vi "loginSession.vi"(8 "error in (no error)":errorcluster, 10 "Device index":i32, 11 "SM1000-control in":T1) -> (0 "error out":errorcluster, 3 "SM1000-control out":T1)   [LabVIEW 2013, in "HardwareCharacterization.lvlib" / "HC-SM1000.lvclass"]
doc: "Connect to an EC device by establishing a session.\n\nOnce EC1000 modules have been identified via the use of the Broadcast API, a communications session can be opened between the client an a selected target EC1000. Sessions are established via a call to this method. Multiple sessions to different target EC1000 controllers are made by instantiating separate Session objects. A target EC1000 controller may only serve one client session at a time."
uses:
  HC-SM1000.lvclass
  Object-reference.ctl
  HC-SM1000.lvclass/HC-SM1000.ctl
  Custom-errors.ctl
  C:/Users/vangeste/Desktop/2015-05-29 - SLM - MAIF/HC-HardwareCharacterization/Sources/SM1000/LECSession.dll
  LECSession.dll
  DOTNET-error-int.vi
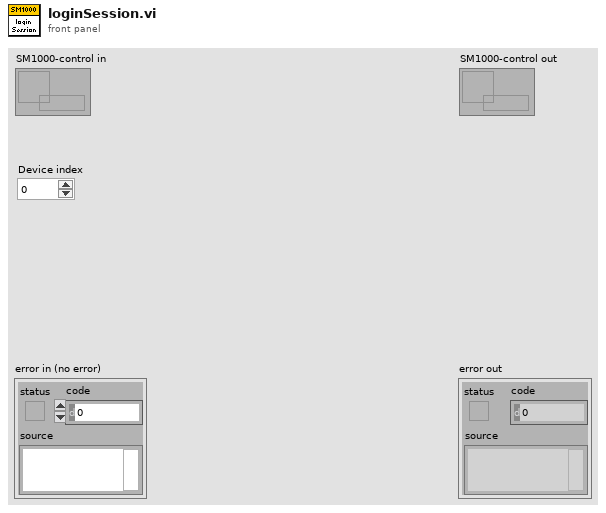
[diagram p1: front panel]
types:
  T1 = typedef "HardwareCharacterization.lvlib/HC-SM1000.lvclass/Object-reference.ctl" = refnum<data-value>
  T2 = typedef "HardwareCharacterization.lvlib/HC-SM1000.lvclass/Custom-errors.ctl" = enum16{"No error", "Not implemented", "Command not recognized", "Invalid input", "No connection", "Timeout", "Resource not loaded"}
  T3 = typedef "HardwareCharacterization.lvlib/HC-SM1000.lvclass/Device-identification.ctl" = cluster{"Name":string, "IP":string, "Mac address":string}
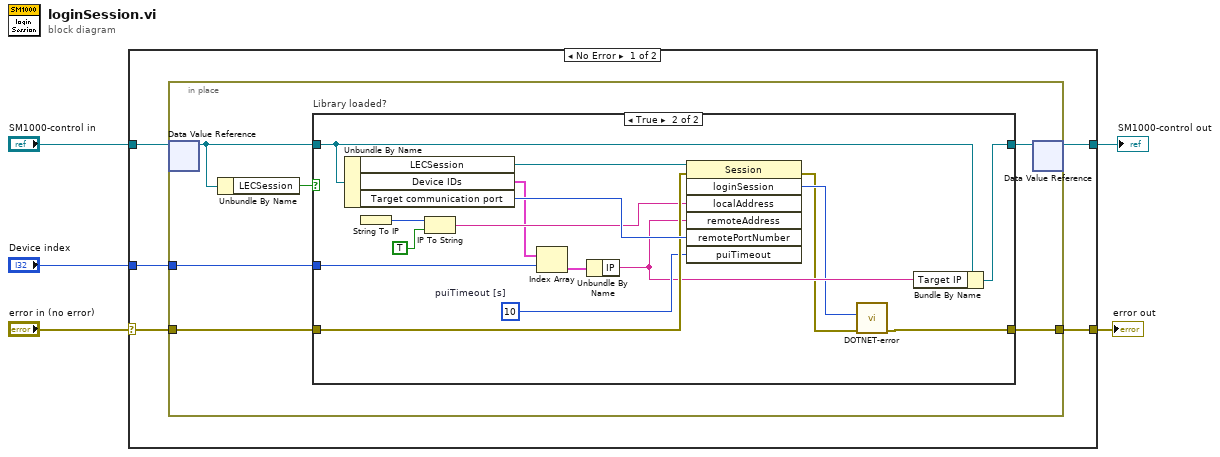
[diagram p0: block diagram]
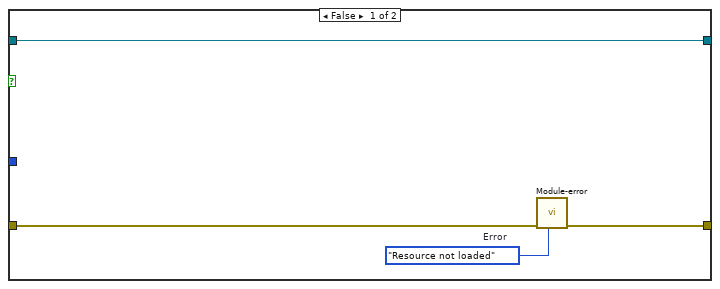
[diagram p2: hidden frame]
diagram:
  n1 = case shown="No Error" "error in (no error)" {
    selector: "error in (no error)" -> [w8 w38]
    tunnel: [w7 w38] -> w4
    tunnel: [w9 w37] -> w2
    tunnel: "SM1000-control in" -> [w10 w37]
    tunnel: "Device index" -> [w6 _]
    frame No Error {
      n2 = in-place {
        in-place-border: w8 -> [w16]
        in-place-border: [w13] -> w7
        in-place-border: w6 -> [w11]
        n3 = in-place-dvr #1(w10) -> (w14:refnum<class "HC-SM1000.lvclass">)  [unwired: 1 out]
        n4 = Unbundle By Name(w14) -> ("LECSession"=w15:bool)
        n5 = case "Library loaded?" shown="True" w15 {
          tunnel: w16 -> [w20 w33]
          tunnel: w14 -> [w18 w31]
          tunnel: [w19 w24] -> w13
          tunnel: [w18 w26] -> w12
          tunnel: w11 -> [_ w29]
          frame False {
            w17 = Custom-errors."Resource not loaded"  # Error
            n6 = call "Module-error.vi"("Error"=w17, "error in (no error)"=w20) -> ("error out"=w19:errorcluster)  [unwired: 9 in]
          }
          frame True {
            w30 = u32 10  # puiTimeout [s]
            n7 = Unbundle By Name(w31) -> ("LECSession"=w35:refnum<k24>, "Device IDs"=w28:T3[], "Target communication port"=w34:i32)
            n8 = String To IP() -> (0:w36:u32)  [unwired: 1 in]
            n9 = IP To String(1:TRUE, 2:w36) -> (0:w32:string)
            n10 = Index Array(array=w28, index=w29) -> (element=w27:T3)
            n11 = Unbundle By Name(w27) -> ("IP"=w25:string)
            n12 = invoke class="Session" method="loginSession"(reference=w35, error in=w33, "localAddress"=w32, "remoteAddress"=w25, "remotePortNumber"=w34, "puiTimeout"=w30) -> (error out=w22:errorcluster, "loginSession"=w23:u32)  [unwired: 1 in, 5 out]
            n13 = call-poly "DOTNET-error.vi"("error in (no error)"=w22, "Retun code"=w23) -> ("error out"=w24:errorcluster)  [unwired: 9 in]
            n14 = Bundle By Name(cluster=w31, "Target IP"=w25) -> (w26:refnum<class "HC-SM1000.lvclass">)
          }
        }
        n15 = in-place-dvr #1(w12) -> (w9:T1)  [unwired: 1 out]
      }
    }
    frame Error {
    }
  }
  "error out" <- w4
  "SM1000-control out" <- w2
